vi "NXTSumoEyes-Dual.vi"() -> ()   [LabVIEW 2009]
uses:
  <vilib>/NXT/Block Support/NXT_InputPort.ctl
  <vilib>/NXT/Subs/LVHSConnector.ctl
  mindsensors.com LVEE Toolkit/Dual/NXTSumoEyes-DM.vi
panel:
  in  "Input of NXTSumoEyes":cluster{"Select Range":u16}={"Select Range"=6} {"Select Range" items=["short"=5, "long"=6]}
  out "NXT dup":T1={"error"={"status"=FALSE, "code"=0, "source"=""}, "address"="", "NXT #"=-1, "Show Error"=TRUE}
  in  "NXT":T1={"error"={"status"=FALSE, "code"=0, "source"=""}, "address"="", "NXT #"=-1, "Show Error"=TRUE}
  in  "Input Port":T2 items=["Port 1", "Port 2", "Port 3", "Port 4"]
  out "Right":bool
  out "Left":bool
  in  "?":bool=TRUE
  # "mindsensors.com\nCopyright (c) 2009 by mindsensors.com\nEmail: info (<at>) mindsensors (<dot>) com\n\nThis program is free software. You can redistribute it and/or modify\nit under the terms of the GNU General Public License as published by\nthe Free Software Foundation; version 3 of the License.\nRead the license at: http://www.gnu.org/licenses/gpl.txt"
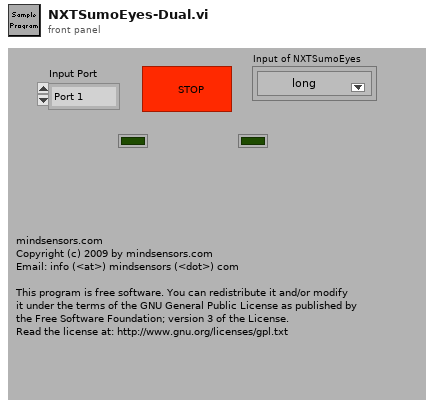
[diagram p1: front panel]
types:
  T1 = typedef "LVHSConnector.ctl" = cluster{"error":errorcluster, "address":string, "NXT #":i32, "Show Error":bool}
  T2 = typedef "NXT_InputPort.ctl" = u8
  T3 = cluster{"Start X":i16, "Start  Y":i16, "Width":i16, "Height":i16}
  T4 = cluster{"Which Zone?":u8, "Scaled Value":i16, "Status":bool}
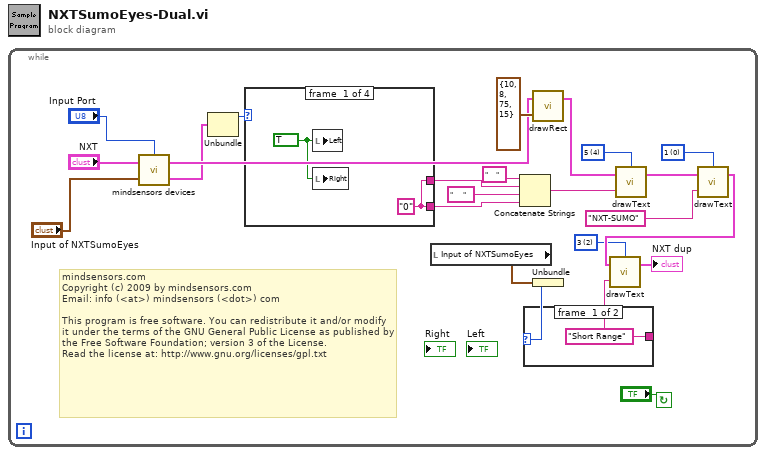
[diagram p0: block diagram]
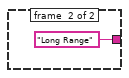
[diagram p2: hidden frame]
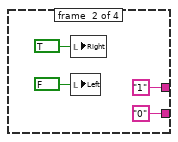
[diagram p3: hidden frame]
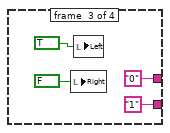
[diagram p4: hidden frame]
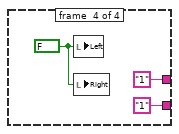
[diagram p5: hidden frame]
diagram:
  n1 = while {
    stop <- "?" continue-if-true
    w6 = i16 2 items=["1", "2", "3", "4", "5", "6", "7", "8"] ("Line")
    w13 = i16 0 items=["1", "2", "3", "4", "5", "6", "7", "8"] ("Line")
    w19 = i16 4 items=["1", "2", "3", "4", "5", "6", "7", "8"] ("Line")
    # "mindsensors.com\nCopyright (c) 2009 by mindsensors.com\nEmail: info (<at>) mindsensors (<dot>) com\n\nThis program is free software. You can redistribute it and/or modify\nit under the terms of the GNU General Public License as published by\nthe Free Software Foundation; version 3 of the License.\nRead the license at: http://www.gnu.org/licenses/gpl.txt"
    n2 = call-poly "mindsensors devices.vi"("Input of NXTSumoEyes"="Input of NXTSumoEyes", "NXT"="NXT", "Input Port"="Input Port") -> ("Output of NXTSumoEyes"=w2:T4, "NXT dup"=w20:T1)
    n3 = Unbundle(w2) -> ("Which Zone?"=w3:u8)  [unwired: 2 out]
    n4 = case shown="3" w3 {
      tunnel: [w27 "1" "0" "1"] -> w11
      tunnel: [w27 "0" "1" "1"] -> w10
      frame #0 {
        w27 = "0"
        w28 = TRUE
        n5 = local write "Left"(w28) -> ()
        n6 = local write "Right"(w28) -> ()
      }
      frame #1 {
        n7 = local write "Right"(TRUE ("Right")) -> ()
        n8 = local write "Left"(FALSE ("Left")) -> ()
      }
      frame #2 {
        n9 = local write "Right"(FALSE ("Right")) -> ()
        n10 = local write "Left"(TRUE ("Left")) -> ()
      }
      frame #3 {
        w37 = FALSE ("Left")
        n11 = local write "Left"(w37) -> ()
        n12 = local write "Right"(w37) -> ()
      }
    }
    n13 = local read "Input of NXTSumoEyes"() -> (w9:cluster{"Select Range":u16})
    n14 = Concatenate Strings("    " ("string"), w11, "     " ("string"), w10) -> (w16:string)
    n15 = call <vilib>:"drawRect.vi"("Rect Parameters"=T3 {"Start X"=10, "Start  Y"=8, "Width"=75, "Height"=15}, "NXT"=w20) -> ("NXT"=w15:T1)  [unwired: 2 in]
    n16 = Unbundle(w9) -> ("Select Range"=w8:u16)
    n17 = case shown="1" w8 {
      tunnel: ["Short Range" "Long Range"] -> w4
      frame #0 {
      }
      frame #1 {
      }
    }
    n18 = call <vilib>:"drawText.vi"("Text"=w16, "NXT"=w15, "Line"=w19) -> ("NXT"=w14:T1)  [unwired: 1 in]
    n19 = call <vilib>:"drawText.vi"("Text"="NXT-SUMO", "NXT"=w14, "Line"=w13) -> ("NXT"=w7:T1)  [unwired: 1 in]
    n20 = call <vilib>:"drawText.vi"("Text"=w4, "NXT"=w7, "Line"=w6) -> ("NXT"=→"NXT dup":T1)  [unwired: 1 in]
  }
